vi "Edit Exchanges.vi"(8 "error in (no error)":errorcluster caption="entrée d'erreur (pas d'erreur)", 9 "Parameters":T1, 10 "Key":i32, 11 "Exchanges en entrée":refnum<class "Exchanges.lvclass"> caption="DNL_LabVIEW Object in") -> (0 "error out":errorcluster caption="sortie d'erreur", 1 "created new?":bool, 3 "Exchanges en sortie":refnum<class "Exchanges.lvclass"> caption="DNL_LabVIEW Object out")   [LabVIEW 2012, in "Exchanges.lvclass"]
uses:
  Exchanges.lvclass
  Exchange/Exchange Parameters.ctl
  Exchange/Exchange Type Enum.ctl
  controls/Currencies.ctl
  <userlib>/_OpenG.lib/dictionary/dictionary.llb/Dictionary Key Value Pair Cluster__ogtk.ctl
  Exchanges.lvclass/Exchanges.ctl
  <userlib>/_OpenG.lib/dictionary/dictionary.llb/Dictionary Update (by scalar value)__ogtk.vi
  Exchange/Exchange.lvclass
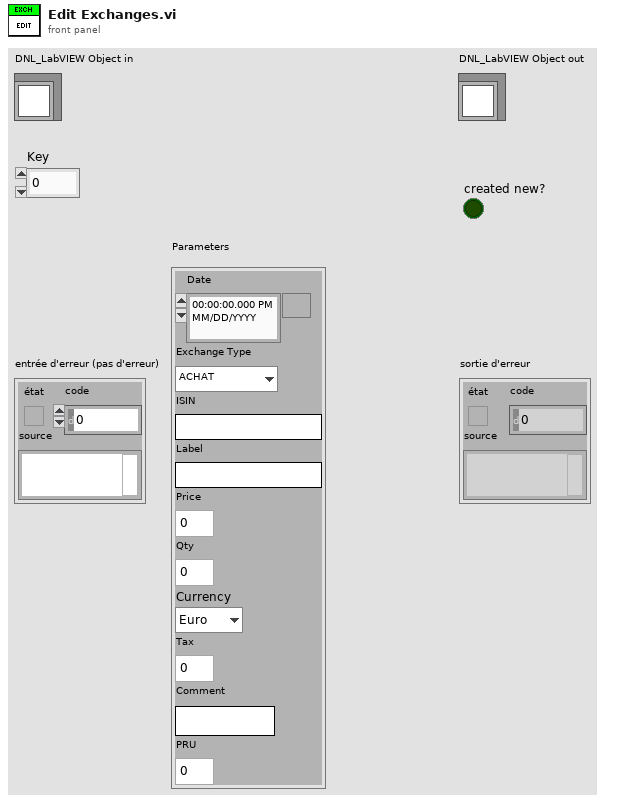
[diagram p1: front panel]
types:
  T1 = typedef "Exchange Parameters.ctl" = cluster{"Date":timestamp, "Exchange Type":T2, "ISIN":string, "Label":string, "Price":dbl, "Qty":dbl, "Currency":T3, "Tax":dbl, "Comment":string, "PRU":dbl}
  T2 = typedef "Exchange.lvclass/Exchange Type Enum.ctl" = enum16{"ACHAT", "VENTE"}
  T3 = typedef "Currencies.ctl" = enum16{"Euro", "Dollar", "Yen", "RIM", "CHF"}
  T4 = typedef "Dictionary Key Value Pair Cluster__ogtk.ctl" = cluster{"key":variant, "value":variant}
  T5 = typedef "Dictionary Object RefNum__ogtk.ctl" = refnum<k1>
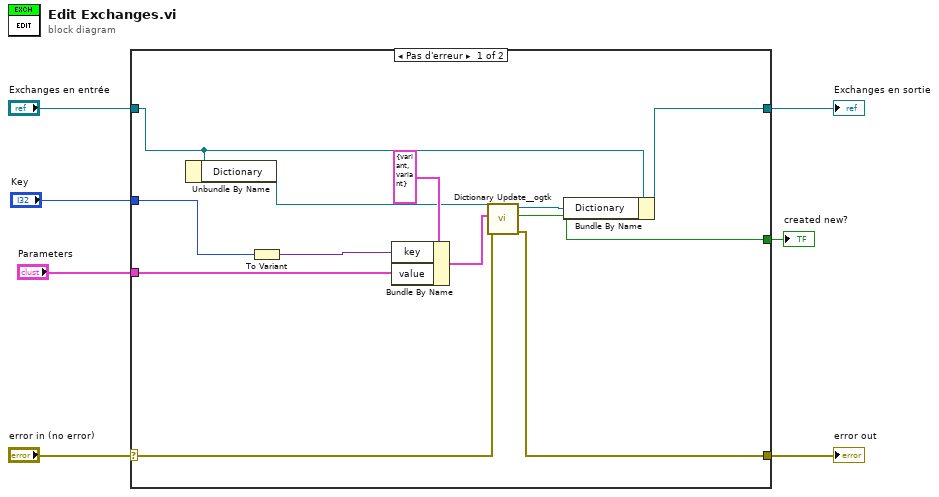
[diagram p0: block diagram]
diagram:
  n1 = case shown="Pas d'erreur" "error in (no error)" {
    selector: "error in (no error)" -> [w11 w21]
    tunnel: [w10 w21] -> w6
    tunnel: [w12 w20] -> w4
    tunnel: "Exchanges en entrée" -> [w13 w20]
    tunnel: [w14 _] -> w3
    tunnel: "Parameters" -> [w9 _]
    tunnel: "Key" -> [w8 _]
    frame No Error {
      n2 = Unbundle By Name(w13) -> ("Dictionary"=w16:T5)
      n3 = To Variant(anything=w8) -> (Variant=w15:variant)
      n4 = Bundle By Name(cluster=T4 {"key"=variant, "value"=variant} ("key-value"), "key"=w15, "value"=w9) -> (w17:T4)
      n5 = call-poly <userlib>:"Dictionary Update__ogtk.vi"("error in (no error)"=w11, "key-value"=w17, "dictionary"=w16) -> ("error out"=w10:errorcluster, "created new?"=w14:bool, "dictionary out"=w19:T5)  [unwired: 6 in]
      n6 = Bundle By Name(cluster=w13, "Dictionary"=w19) -> (w12:refnum<class "Exchanges.lvclass">)
    }
    frame Error {
    }
  }
  "error out" <- w6
  "Exchanges en sortie" <- w4
  "created new?" <- w3
